vi "MemoryGlobal.vi"(7 "Action":T1, 11 "Set Value":string[](array[string])) -> (3 "Value Out":string[](array[string]))   [LabVIEW 2012]
uses:
  MemoryGlobalAction.ctl
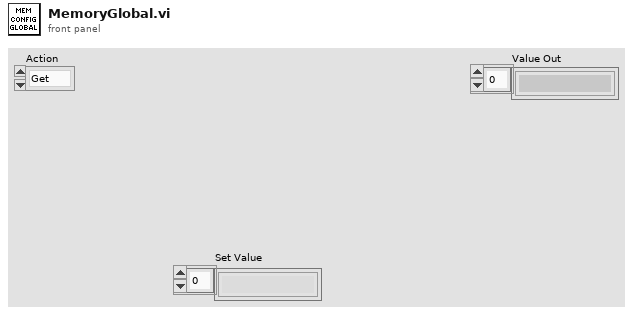
[diagram p1: front panel]
types:
  T1 = typedef "MemoryGlobalAction.ctl" = enum16{"Get", "Set", "Reset"}
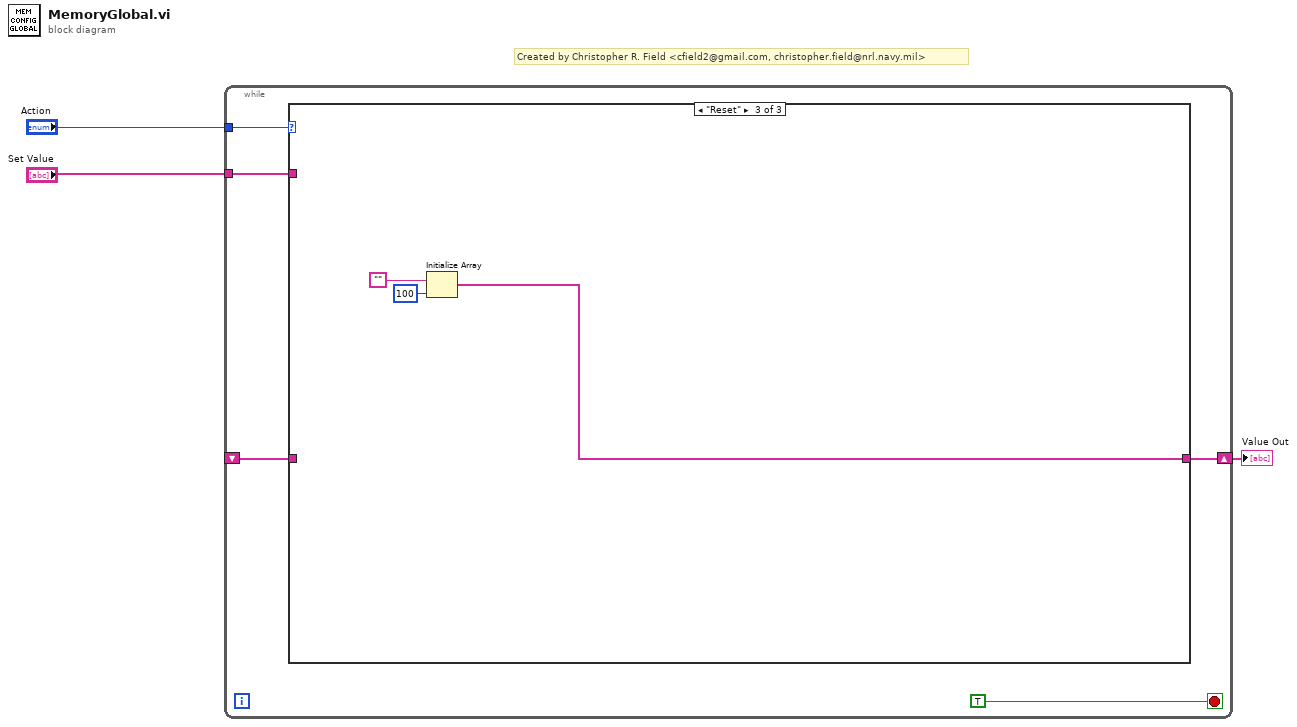
[diagram p0: block diagram]
diagram:
  # "Created by Christopher R. Field <cfield2@gmail.com, christopher.field@nrl.navy.mil>"
  n1 = while {
    tunnel: "Action" -> [w7]
    shift-right: [w6] -> w1
    shift-left: _ -> [w5]
    tunnel: "Set Value" -> [w4]
    stop <- TRUE stop-if-true
    n2 = case shown="\"Reset\"" w7 {
      tunnel: [w9 w10 w11] -> w6
      tunnel: w5 -> [w9 _ _]
      tunnel: w4 -> [_ w10 _]
      frame "Get", Default {
      }
      frame "Set" {
      }
      frame "Reset" {
        n3 = Initialize Array("", 100 ("dimension size")) -> (w11:string[])
      }
    }
  }
  "Value Out" <- w1
